vi "K24xx Vsweep Coarse.vi"(5 "Time Interval (sec)":dbl=0.5 min=0.1 step=0.1, 6 "stop":bool, 7 "Sweep Time (H:M:S)":dbl=3600.0 format="%<%H:%M:%S>t", 8 "Mapping":bool, 9 "End Voltage (V)":dbl=1e-10 format="%.3e", 10 "Start Voltage (V)":dbl=1e-06 format="%.3e", 11 "Keithley 24XX Address":refnum<visa-resource-name>) -> (1 "Last Sent Value":dbl=1e-06 format="%.3e")   [LabVIEW 2024]
uses:
  Global Variables/Voltage K24xx Coarse.vi
panel:
  out "Prepared Value":dbl=1e-06 format="%.3e"
  out "Iteration":i32
  # "Add two extra sec for timing."
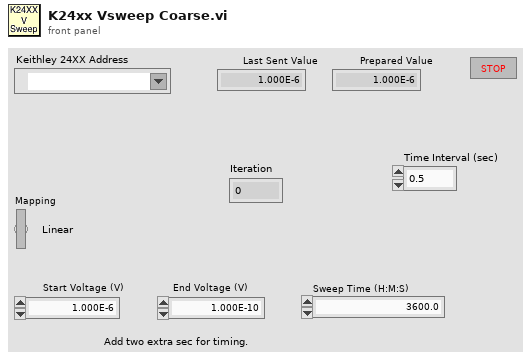
[diagram p1: front panel]
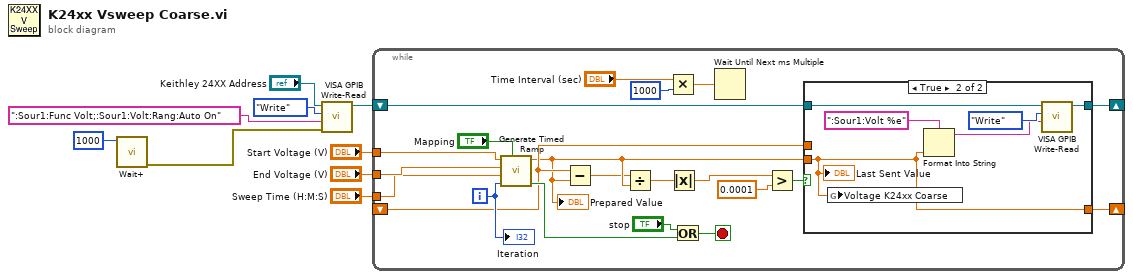
[diagram p0: block diagram]
diagram:
  n1 = call "Wait+.vi"("milliseconds to wait"=u32 1000) -> ("Error Out"=w8:errorcluster)  [unwired: 5 in, 1 out]
  n2 = call "VISA GPIB Write-Read.vi"("error in (no error)"=w8, "Command"=":Sour1:Func Volt;:Sour1:Volt:Rang:Auto On", "Action"=enum16{"Write", "Read", "Write & Read"}."Write", "VISA resource name"="Keithley 24XX Address") -> ("dup VISA Session"=w3:refnum<visa-resource-name>)  [unwired: 4 in, 3 out]
  n3 = while {
    tunnel: "Start Voltage (V)" -> [w30]
    tunnel: "End Voltage (V)" -> [w29]
    tunnel: "Sweep Time (H:M:S)" -> [w28]
    shift-right: [w21] -> _
    shift-left: _ -> [w19]
    shift-right: [w10] -> _
    shift-left: w3 -> [w17]
    i -> [w27]
    stop <- w25 stop-if-true
    n4 = call "Generate Timed Ramp.vi"("Log"="Mapping", "Point #"=w27, "Time (Hr:Min:Sec)"=w28, "Stop"=w29, "Start"=w30) -> ("Stop"=w24:bool, "Output"=w18:dbl)  [unwired: 2 out]
    "Prepared Value" <- w18
    n5 = Subtract(x=w19, y=w18) -> (x-y=w13:dbl)
    n6 = Divide(x=w13, y=w18) -> (x/y=w12:dbl)
    n7 = Multiply(x="Time Interval (sec)", y=u32 1000 ("millisecond multiple")) -> (x*y=w15:dbl)
    n8 = Absolute Value(x=w12) -> (abs(x)=w11:dbl)
    n9 = Or(x="stop", y=w24) -> (x .or. y?=w25:bool)
    n10 = Wait Until Next ms Multiple(millisecond multiple=w15) -> ()  [unwired: 1 out]
    n11 = Greater?(x=w11, y=0.0001) -> (0:w20:bool)
    n12 = case shown="True" w20 {
      tunnel: [w32 w34] -> w21
      tunnel: w19 -> [w32 _]
      tunnel: w18 -> [_ w34]
      tunnel: w17 -> [w31 w38]
      tunnel: [w31 w35] -> w10
      frame False {
      }
      frame True {
        n13 = global write "Voltage K24xx Coarse.vi" "Voltage K24xx Coarse"(w34) -> ()
        n14 = Format Into String(format string=":Sour1:Volt %e", w34) -> (resulting string=w36:string)  [unwired: 2 in, 1 out]
        n15 = call "VISA GPIB Write-Read.vi"("Command"=w36, "Action"=enum16{"Write", "Read", "Write & Read"}."Write", "VISA resource name"=w38) -> ("dup VISA Session"=w35:refnum<visa-resource-name>)  [unwired: 5 in, 3 out]
        "Last Sent Value" <- w34
      }
    }
    "Iteration" <- w27
  }
